vi "Sixtypes Insert.vi"() -> ()   [LabVIEW 2018]
doc: "This VI shows how you can insert data of different data types into a table named sixtypes in the LabVIEW.mdb database. \n\nThe table is deleted if it already exists. A new table is created using the column names and data types defined by the column information array on the panel. The values shown at the bottom of the panel are the ones actually inserted into the table fields.\n\nYou can use the Sixtypes Select VI to read the values back from the table."
uses:
  <vilib>/addons/database/Auxilliary.llb/DB Tools Column Info.ctl
  <vilib>/addons/database/Auxilliary.llb/DB Tools DataTypes.ctl
  <vilib>/addons/database/Connection.llb/DB Tools Open Connec (Path).vi
  <vilib>/addons/database/Auxilliary.llb/DB Tools Format Datetime String (Time Stamp).vi
  <vilib>/addons/database/NI_Database_API.lvlib
panel:
  out "Date/Time":string
  in  "Numeric (CDB)":cdb=12.5-98.04i format="%.2f"
  in  "Numeric (DBL)":dbl=1202.556
  in  "Numeric (SGL)":sgl=-0.02168
  in  "Numeric (I32)":i32=125
  in  "String":string="this is a test."
  in  "column information":T1[](array[typedef])=[{"column name"="Str", "data type"=enum."String", "size"=30, "allow null?"=FALSE}, {"column name"="I32", "data type"=enum."Long (I32)", "size"=0, "allow null?"=FALSE}, {"column name"="SGL", "data type"=enum."Single (SGL)", "size"=0, "allow null?"=FALSE}, {"column name"="DBL", "data type"=enum."Double (DBL)", "size"=0, "allow null?"=FALSE}, {"column name"="DT", "data type"=enum."Date/Time", "size"=0, "allow null?"=FALSE}, {"column name"="Bin", "data type"=enum."Binary", "size"=0, "allow null?"=FALSE}]
  # "Overview: Demonstrates how to insert various data types into a table in a database.\nRequirements: Database Connectivity Toolkit\nInstructions:\nRun the VI. All six data types are inserted into the table."
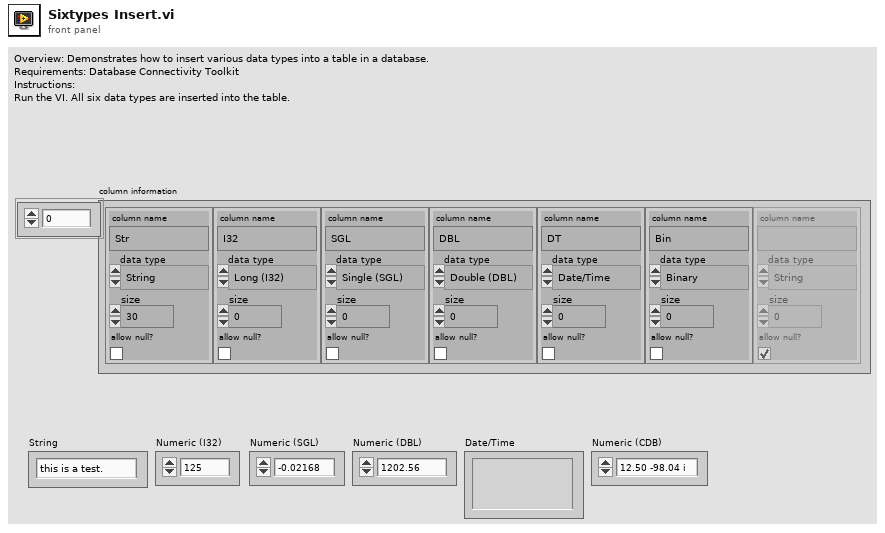
[diagram p1: front panel]
types:
  T1 = typedef "NI_Database_API.lvlib/DB Tools Column Info.ctl" = cluster{"column name":string, "data type":T2, "size":i32, "allow null?":bool}
  T2 = typedef "NI_Database_API.lvlib/DB Tools DataTypes.ctl" = enum16{"String", "Long (I32)", "Single (SGL)", "Double (DBL)", "Date/Time", "Binary"}
  T3 = typedef "NI_Database_API.lvlib/Conn ObjectReference.ctl" = refnum<k1>
  T4 = cluster{"String":string, "Numeric (I32)":i32, "Numeric (SGL)":sgl, "Numeric (DBL)":dbl, "date/time string":string, "Numeric (CDB)":cdb}
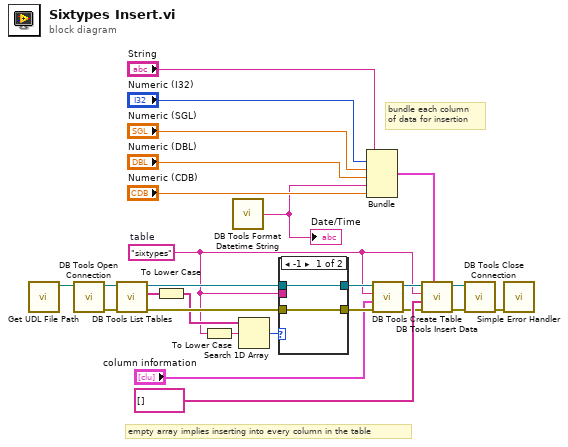
[diagram p0: block diagram]
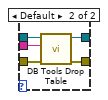
[diagram p2: hidden frame]
diagram:
  w4 = "sixtypes"  # table
  # "bundle each column\nof data for insertion"
  # "empty array implies inserting into every column in the table"
  n1 = call "Get UDL File Path.vi"() -> ("UDL file path"=w2:path)  [unwired: 11 in]
  n2 = call-poly <vilib>:"DB Tools Open Connection.vi"("connection information"=w2) -> ("error out"=w26:errorcluster, "connection reference"=w25:T3)  [unwired: 7 in]
  n3 = call <vilib>:"DB Tools List Tables.vi"("error in (no error)"=w26, "connection reference"=w25) -> ("error out"=w23:errorcluster, "tables"=w24:string[], "connection reference out"=w22:T3)  [unwired: 3 in]
  n4 = To Lower Case(string=w24) -> (all lower case string=w21:string[])
  n5 = To Lower Case(string=w4) -> (all lower case string=w20:string)
  n6 = call-poly <vilib>:"DB Tools Format Datetime String.vi"() -> ("date/time string"=w1:string)  [unwired: 1 in]
  "Date/Time" <- w1
  n7 = Search 1D Array(1D array=w21, element=w20) -> (index of element=w19:i32)  [unwired: 1 in]
  n8 = case shown="-1" w19 {
    tunnel: w23 -> [w27 w33]
    tunnel: w22 -> [w28 w32]
    tunnel: [w28 w31] -> w8
    tunnel: [w27 w30] -> w9
    tunnel: w4 -> [_ w29]
    frame -1 {
    }
    frame Default {
      n9 = call <vilib>:"DB Tools Drop Table.vi"("error in (no error)"=w33, "table"=w29, "connection reference"=w32) -> ("error out"=w30:errorcluster, "connection reference out"=w31:T3)  [unwired: 5 in]
    }
  }
  n10 = Bundle("String"="String", "Numeric (I32)"="Numeric (I32)", "Numeric (SGL)"="Numeric (SGL)", "Numeric (DBL)"="Numeric (DBL)", "date/time string"=w1, "Numeric (CDB)"="Numeric (CDB)") -> (w10:T4)  [unwired: 1 in]
  n11 = call <vilib>:"DB Tools Create Table.vi"("error in (no error)"=w9, "column information"="column information", "table"=w4, "connection reference"=w8) -> ("error out"=w6:errorcluster, "connection reference out"=w7:T3)  [unwired: 4 in]
  n12 = call <vilib>:"DB Tools Insert Data.vi"("data"=w10, "error in (no error)"=w6, "columns"=string[] [], "table"=w4, "connection reference"=w7) -> ("error out"=w17:errorcluster, "connection reference out"=w16:T3)  [unwired: 5 in]
  n13 = call <vilib>:"DB Tools Close Connection.vi"("error in (no error)"=w17, "connection reference"=w16) -> ("error out"=w3:errorcluster)  [unwired: 5 in]
  n14 = call <vilib>:"Simple Error Handler.vi"("error in (no error)"=w3) -> ()  [unwired: 4 in, 5 out]
